vi "Application Folder.vi"(3 "Relative Path (\"\" - Folder)":string) -> (1 "Application Folder":path)   [LabVIEW 2011]
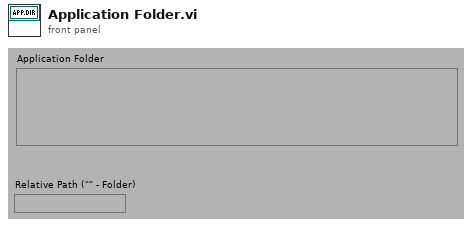
[diagram p1: front panel]
types:
  T1 = enum32{"invalid app kind", "Development System", "Run Time System", "Student Edition", "Embedded LabVIEW", "Evaluation", "Custom"}
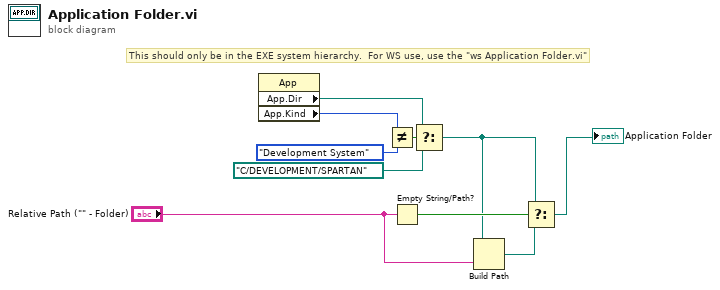
[diagram p0: block diagram]
diagram:
  # "This should only be in the EXE system hierarchy.  For WS use, use the \"ws Application Folder.vi\""
  n1 = property class="App"() -> ("App.Dir"=w4:path, "App.Kind"=w2:T1)  [unwired: 2 in, 2 out]
  n2 = Not Equal?(x=w2, y=T1."Development System") -> (x != y?=w5:bool)
  n3 = Empty String/Path?(string/path="Relative Path (\"\" - Folder)") -> (empty?=w8:bool)
  n4 = Select(t=w4, s=w5, f=path "C:/DEVELOPMENT/SPARTAN" ("start path")) -> (s? t:f=w3:path)
  n5 = Build Path(base path=w3, name or relative path="Relative Path (\"\" - Folder)") -> (appended path=w7:path)
  n6 = Select(t=w3, s=w8, f=w7) -> (s? t:f=→"Application Folder":path)
